vi "RSZVB Shift Limit Line Segment List.vi"(6 "Stimulus Offset (0.0)":dbl format="%^.3e", 7 "Response Offset (0.0)":dbl format="%^.3e", 8 "error in (no error)":errorcluster {"code" format="%.0x"}, 9 "Limit Line Type (2: Upper)":i32(ring)=2 items=["Lower"=2, "Upper"=1], 10 "Channel (Trace) (1)":i32=1, 11 "VISA session":refnum<visa-resource-name>) -> (0 "error out":errorcluster {"code" format="%.0x"}, 3 "dup VISA session":refnum<visa-resource-name>)   [LabVIEW 2011]
doc: "This VI shifts the limit line in horizontal direction (stimulus values) and also shifts all lower and upper limit line segments assigned to the active trace in vertical direction (response values).\n\nRemote-control command(s):\nCALCulate<Ch/Tr>:LIMit:CONTrol:SHIFt <numeric_value>\nCALCulate<Ch/Tr>:LIMit:LOWer:SHIFt <numeric_value>\nCALCulate<Ch/Tr>:LIMit:UPPer:SHIFt <numeric_value>"
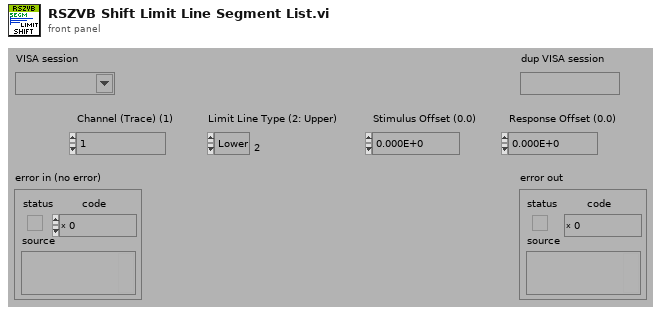
[diagram p1: front panel]
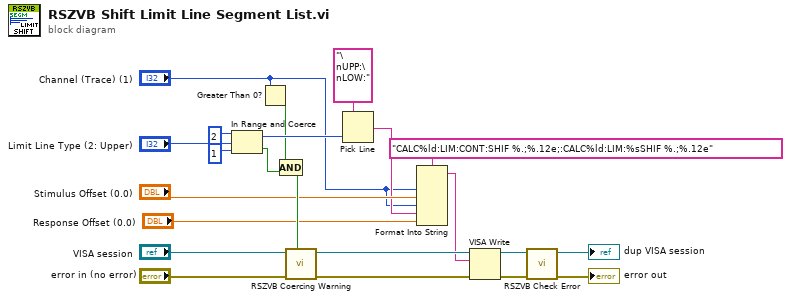
[diagram p0: block diagram]
diagram:
  n1 = In Range and Coerce(upper limit=2, x="Limit Line Type (2: Upper)", lower limit=1) -> (coerced(x)=w3:i32, In Range?=w15:bool)
  n2 = Greater Than 0?(x="Channel (Trace) (1)") -> (x > 0?=w1:bool)
  n3 = Compound Arithmetic op=AND(w1, w15) -> (w14:bool)
  n4 = call "RSZVB Coercing Warning.vi"("In Range?"=w14, "error in (no error)"="error in (no error)", "VISA session"="VISA session") -> ("error out"=w21:errorcluster, "dup VISA session"=w22:refnum<visa-resource-name>)  [unwired: 7 in]
  n5 = Pick Line(multi-line string="\nUPP:\nLOW:", line index=w3) -> (output string=w5:string)  [unwired: 1 in]
  n6 = Format Into String(format string="CALC%ld:LIM:CONT:SHIF %.;%.12e;:CALC%ld:LIM:%sSHIF %.;%.12e", "Channel (Trace) (1)", "Stimulus Offset (0.0)", "Channel (Trace) (1)", w5, "Response Offset (0.0)") -> (resulting string=w13:string)  [unwired: 2 in, 1 out]
  n7 = VISA Write(VISA resource name=w22, write buffer=w13, error in (no error)=w21) -> (VISA resource name out=w19:refnum<visa-resource-name>, error out=w20:errorcluster)  [unwired: 1 out]
  n8 = call "RSZVB Check Error.vi"("error in (no error)"=w20, "VISA session"=w19) -> ("error out"=→"error out":errorcluster, "dup VISA session"=→"dup VISA session":refnum<visa-resource-name>)  [unwired: 8 in]
